vi "Initialize Reference Range Controller.vi"(8 "error in (no error)":errorcluster, 10 "Settings":T1, 11 "MWWL Verification in":refnum<class "MWWL Verification.lvclass">) -> (0 "error out":errorcluster, 3 "MWWL Verification out":refnum<class "MWWL Verification.lvclass">)   [LabVIEW 2018, in "MWWL Verification.lvlib" / "MWWL Verification.lvclass"]
uses:
  MWWL Verification.lvclass
  C:/Program Files (x86)/National Instruments/LabVIEW 2018/vi.lib/ActorFramework/Actor/Actor.lvclass
  Type Defs/ConfigSettings.ctl
  Range Controller Actor/Range Controller Actor.lvclass
  MWWL Verification.lvclass/MWWL Verification.ctl
  <vilib>/ActorFramework/Actor/Actor.lvclass
  Range Controller Actor/Range Controller Actor Messages/Initialize Range Controller Msg/Initialize Range Controller Msg.lvclass
  MWWL Verification.lvlib
panel:
  # "SM140"
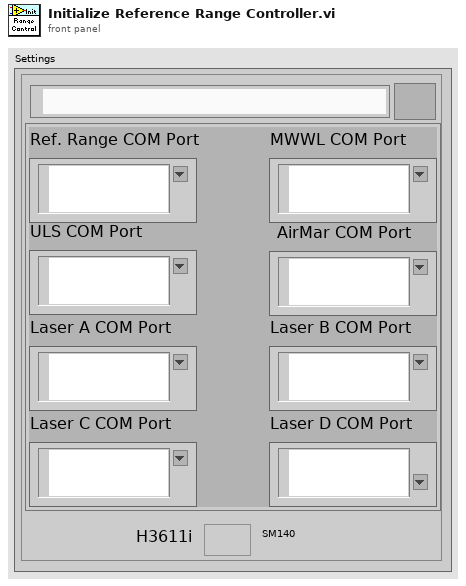
[diagram p1: front panel]
types:
  T1 = typedef "MWWL Verification.lvlib/ConfigSettings.ctl" = cluster{"Base Path":path, "DNL_Configuration Settings.Ports":cluster{"Ref. Range COM Port":refnum<visa-resource-name>, "MWWL COM Port":refnum<visa-resource-name>, "ULS COM Port":refnum<visa-resource-name>, "Laser A COM Port":refnum<visa-resource-name>, "Laser B COM Port":refnum<visa-resource-name>, "Laser C COM Port":refnum<visa-resource-name>, "Laser D COM Port":refnum<visa-resource-name>, "AirMar COM Port":refnum<visa-resource-name>}, "H3611i":bool}
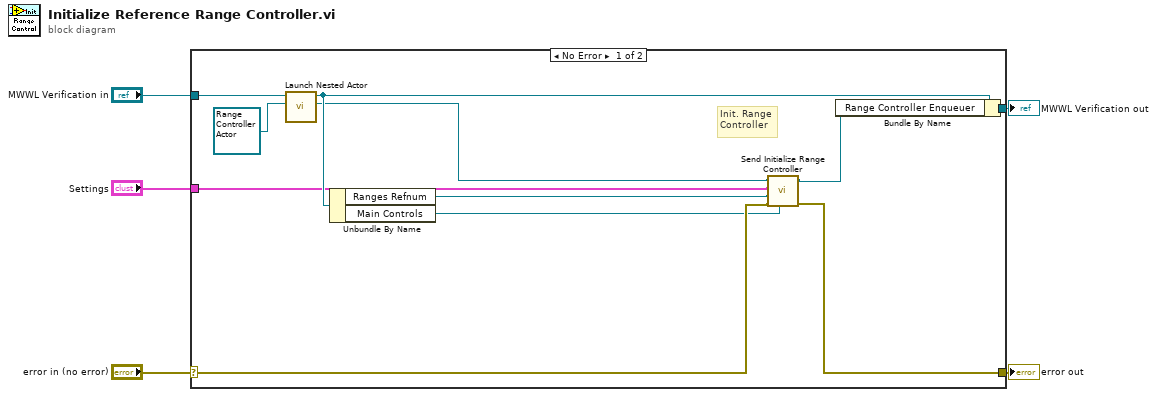
[diagram p0: block diagram]
diagram:
  n1 = case shown="No Error" "error in (no error)" {
    selector: "error in (no error)" -> [w9 w18]
    tunnel: [w10 w18] -> w4
    tunnel: [w15 w17] -> w2
    tunnel: "MWWL Verification in" -> [w16 w17]
    tunnel: "Settings" -> [w7 _]
    frame No Error {
      # "Init. Range\nController"
      n2 = call <vilib>:"Launch Nested Actor.vi"("Nested Actor"=refnum<class "Range Controller Actor.lvclass"> refnum ("Range Controller.lvlib:Range Controller Actor"), "Caller Actor in"=w16) -> ("Nested Actor's Enqueuer"=w12:refnum<class "Message Enqueuer.lvclass">, "Caller Actor out"=w13:refnum<class "MWWL Verification.lvclass">)  [unwired: 7 in, 1 out]
      n3 = Unbundle By Name(w13) -> ("Ranges Refnum"=w8:refnum<vi>, "Main Controls"=w6:refnum<vi>)
      n4 = call "Send Initialize Range Controller.vi"("Main Controls"=w6, "error in (no error)"=w9, "Ranges Refnum"=w8, "Settings"=w7, "Message Enqueuer in"=w12) -> ("error out"=w10:errorcluster, "Message Enqueuer out"=w11:refnum<class "Message Enqueuer.lvclass">)  [unwired: 5 in]
      n5 = Bundle By Name(cluster=w13, "Range Controller Enqueuer"=w11) -> (w15:refnum<class "MWWL Verification.lvclass">)
    }
    frame Error {
    }
  }
  "error out" <- w4
  "MWWL Verification out" <- w2
